vi "DestroySubpanelReference.vi"(8 "error in (no error)":errorcluster, 11 "EmbeddedMainUI in":refnum<class "EmbeddedMainUI.lvclass">) -> (0 "error out":errorcluster, 3 "EmbeddedMainUI out":refnum<class "EmbeddedMainUI.lvclass">)   [LabVIEW 2016, in "EmbeddedMainUI.lvclass"]
uses:
  EmbeddedMainUI.lvclass
  EmbeddedMainUI.lvclass/EmbeddedMainUI.ctl
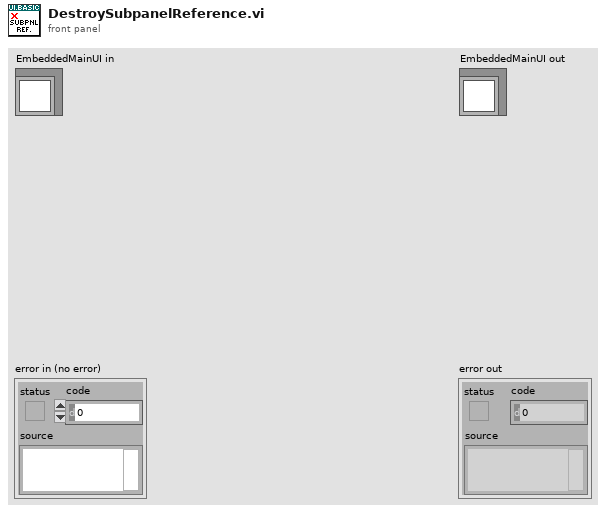
[diagram p1: front panel]
types:
  T1 = typedef "EmbeddedMainUI.lvclass/FrameworkDataRef.ctl" = refnum<data-value>
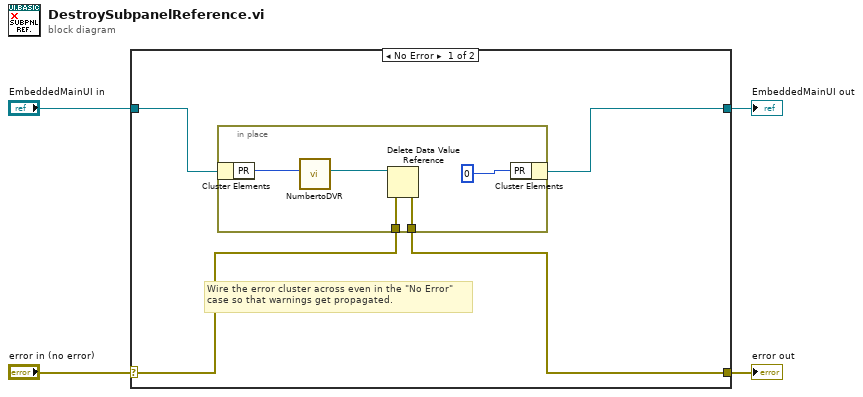
[diagram p0: block diagram]
diagram:
  n1 = case shown="No Error" "error in (no error)" {
    selector: "error in (no error)" -> [w8 w15]
    tunnel: [w7 w15] -> w3
    tunnel: [w5 w14] -> w1
    tunnel: "EmbeddedMainUI in" -> [w6 w14]
    frame No Error {
      # "Wire the error cluster across even in the \"No Error\"\ncase so that warnings get propagated."
      n2 = in-place {
        in-place-border: w8 -> [w13]
        in-place-border: [w12] -> w7
        n3 = in-place-cluster #1(w6) -> ("PR"=w10:i32)
        n4 = call "NumbertoDVR.vi"("Numeric"=w10) -> ("FrameworkDataRef"=w11:T1)  [unwired: 10 in]
        n5 = Delete Data Value Reference(data value reference=w11, error in=w13) -> (error out=w12:errorcluster)  [unwired: 1 out]
        n6 = in-place-cluster #1("PR"=0) -> (w5:refnum<class "EmbeddedMainUI.lvclass">)
      }
    }
    frame Error {
    }
  }
  "error out" <- w3
  "EmbeddedMainUI out" <- w1
